vi "stop.vi"(8 "error in (no error)":errorcluster, 11 "Imaging in":refnum<class "Imaging.lvclass">) -> (0 "error out":errorcluster, 3 "Imaging out":refnum<class "Imaging.lvclass">)   [LabVIEW 2014, in "Imaging.lvclass"]
uses:
  Imaging.lvclass
  Imaging.lvclass/Imaging.ctl
  <vilib>/vision/driver/NI_Vision_Acquisition_Software.lvlib
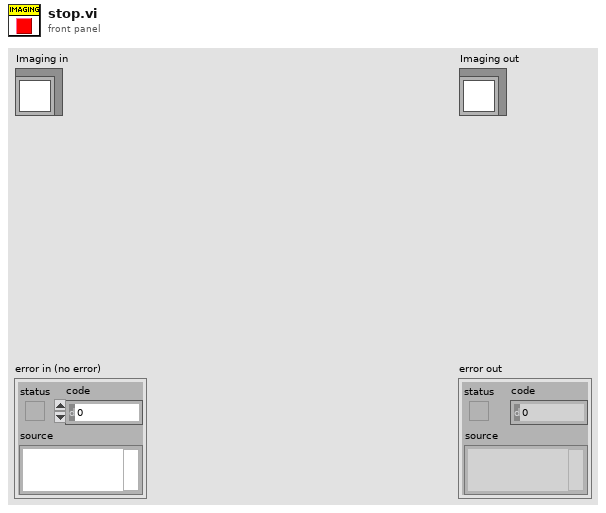
[diagram p1: front panel]
types:
  T1 = typedef "IMAQ Image.ctl" = refnum<image>
  T2 = typedef "IMAQdx.ctl" = refnum<k21>
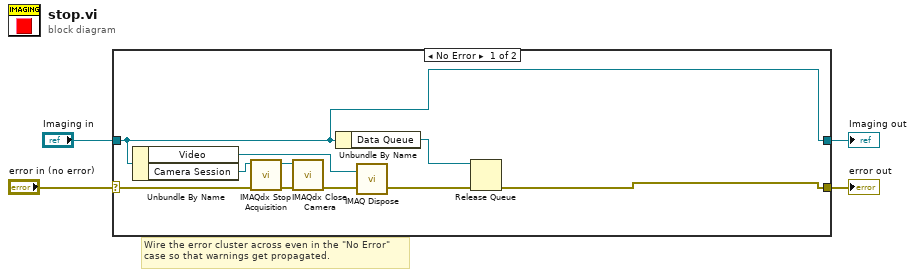
[diagram p0: block diagram]
diagram:
  # "Wire the error cluster across even in the \"No Error\"\ncase so that warnings get propagated."
  n1 = case shown="No Error" "error in (no error)" {
    selector: "error in (no error)" -> [w11 w16]
    tunnel: [w5 w16] -> w3
    tunnel: [w6 w15] -> w1
    tunnel: "Imaging in" -> [w6 w15]
    frame No Error {
      n2 = Unbundle By Name(w6) -> ("Video"=w9:T1, "Camera Session"=w12:T2)
      n3 = call <vilib>:"IMAQdx Stop Acquisition.vi"("error in"=w11, "Session In"=w12) -> ("error out"=w14:errorcluster, "Session Out"=w13:T2)  [unwired: 8 in]
      n4 = call <vilib>:"IMAQdx Close Camera.vi"("error in"=w14, "Session In"=w13) -> ("error out"=w10:errorcluster)  [unwired: 9 in]
      n5 = Unbundle By Name(w6) -> ("Data Queue"=w7:refnum<queue>)
      n6 = call "IMAQ Dispose"("Image"=w9, "error in (no error)"=w10) -> ("error out"=w8:errorcluster)  [unwired: 4 in]
      n7 = Release Queue(queue=w7, error in (no error)=w8) -> (error out=w5:errorcluster)  [unwired: 1 in, 2 out]
    }
    frame Error {
    }
  }
  "error out" <- w3
  "Imaging out" <- w1
